vi "Init Slam.vi"   [LabVIEW 2017]
uses:
  control/Control Globals.vi
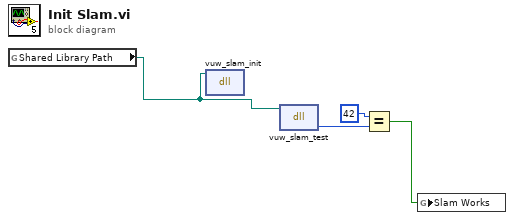
[diagram p0: block diagram]
diagram:
  n1 = global read "Control Globals.vi" "Shared Library Path"() -> (w3:path)
  n2 = dll-call lib="home/admin/lib/libslam.so" fn="vuw_slam_init"(path in=w3) -> ()  [unwired: 3 in, 2 out]
  n3 = dll-call lib="home/admin/lib/libslam.so" fn="vuw_slam_test"(path in=w3) -> ("return type"=w1:i32)  [unwired: 2 in, 2 out]
  n4 = Equal?(x=42, y=w1) -> (x = y?=w4:bool)
  n5 = global write "Control Globals.vi" "Slam Works"(w4) -> ()
